vi "test.vi"() -> ()   [LabVIEW 2018]
doc: "This example demonstrates how to continuously acquire buffered voltage measurements using a DAQmx device.\n\nFor instructions on how to connect your signals to the DAQ device, refer to your device documentation."
uses:
  <vilib>/Utility/error.llb/DialogType.ctl
  <vilib>/DAQmx/read.llb/DAQmx Read (Analog 2D DBL NChan NSamp).vi
  <vilib>/Analysis/baseanly.llb/Mean (DBL).vi
  <vilib>/DAQmx/create/channels.llb/DAQmx Create Channel (AI-Voltage-Basic).vi
  <vilib>/DAQmx/configure/timing.llb/DAQmx Timing (Sample Clock).vi
  <vilib>/DAQmx/configure/task.llb/DAQmx Configure Logging (TDMS).vi
  <vilib>/DAQmx/configure/trigger.llb/DAQmx Start Trigger (Digital Edge).vi
  <vilib>/DAQmx/configure/trigger.llb/DAQmx Start Trigger (Time).vi
  <vilib>/DAQmx/configure/trigger.llb/DAQmx Start Trigger (Analog Edge).vi
  <vilib>/DAQmx/miscellaneous.llb/DAQmx Fill In Error Info.vi
  <resource>/objmgr/daqmx.rc
  <vilib>/Analysis/NI_AALBase.lvlib
panel:
  out "Numeric":i32
  out "Numeric 2":i32
  in  "SAVE":bool
  in  "Path":path
  in  "Name File":string
  in  "Trigger Type":T1(tab)=enum."Digital Start"
  in  "Digital Start Trigger Edge":i32(ring)=10280 caption="Edge" items=["Rising"=10280, "Falling"=10171]
  in  "Digital Start Trigger Source":tag="/Dev2/PFI0" caption="Source"
  in  "Digital Pause Trigger Pause When":i32(ring)=10192 caption="Pause When" items=["High"=10192, "Low"=10214]
  in  "Digital Pause Trigger Source":tag="/Dev1/PFI0" caption="Source"
  in  "Analog Start Trigger Level":dbl caption="Level" format="%0.2f"
  in  "Analog Start Trigger Hysteresis":dbl caption="Hysteresis" format="%.2f"
  in  "Analog Start Trigger Slope":i32(ring)=10280 caption="Slope" items=["Rising"=10280, "Falling"=10171]
  in  "Analog Start Trigger Source":string="APFI0" caption="Source"
  in  "Analog Pause Trigger Source":string="APFI0" caption="Source"
  in  "Analog Pause Trigger Pause When":i32(ring)=10093 caption="Pause When" items=["Above Level"=10093, "Below Level"=10107]
  in  "Analog Pause Trigger Level":dbl caption="Level" format="%.2f"
  in  "When":timestamp
  in  "Select Time\nManually":bool
  in  "SENSOR":bool
  out "Waveform Graph":dbl[][](graph)
  in  "TDMS File Path":path
  in  "Number of Samples":i32=100
  in  "Sample Rate":dbl=10000.0
  in  "Sample Clock Source":tag="OnboardClock"
  in  "Terminal Configuration":i32(ring)=10083 items=["default"=-1, "RSE"=10083, "NRSE"=10078, "Differential"=10106, "Pseudodifferential"=12529]
  in  "Max Voltage":dbl=10.0
  in  "Min Voltage":dbl=-10.0
  in  "Physical Channel":tag="Dev2/ai3:4"
  out "Actual Sample Rate":dbl=1000.0 format="%0.2f"
  in  "Logging Mode":i32(ring)=10231 items=["Off"=10231, "Log and Read"=15842]
  # "Channel Settings"
  # "Acquired Data"
  # "Timing Settings"
  # "Logging Settings"
  # "Trigger Settings"
  # "To enable triggers, select a tab above, and configure the settings.\n\nNot all hardware supports all trigger types. Refer to your device documentation for more information."
  # "This trigger type is not supported in continuous sample timing. \n\nRefer to your device documentation for more information on which triggers are supported."
  # "This trigger type is not supported in continuous sample timing. \n\nRefer to your device documentation for more information on which triggers are supported."
  # "If time is not manually set, task will begin after 10 seconds"
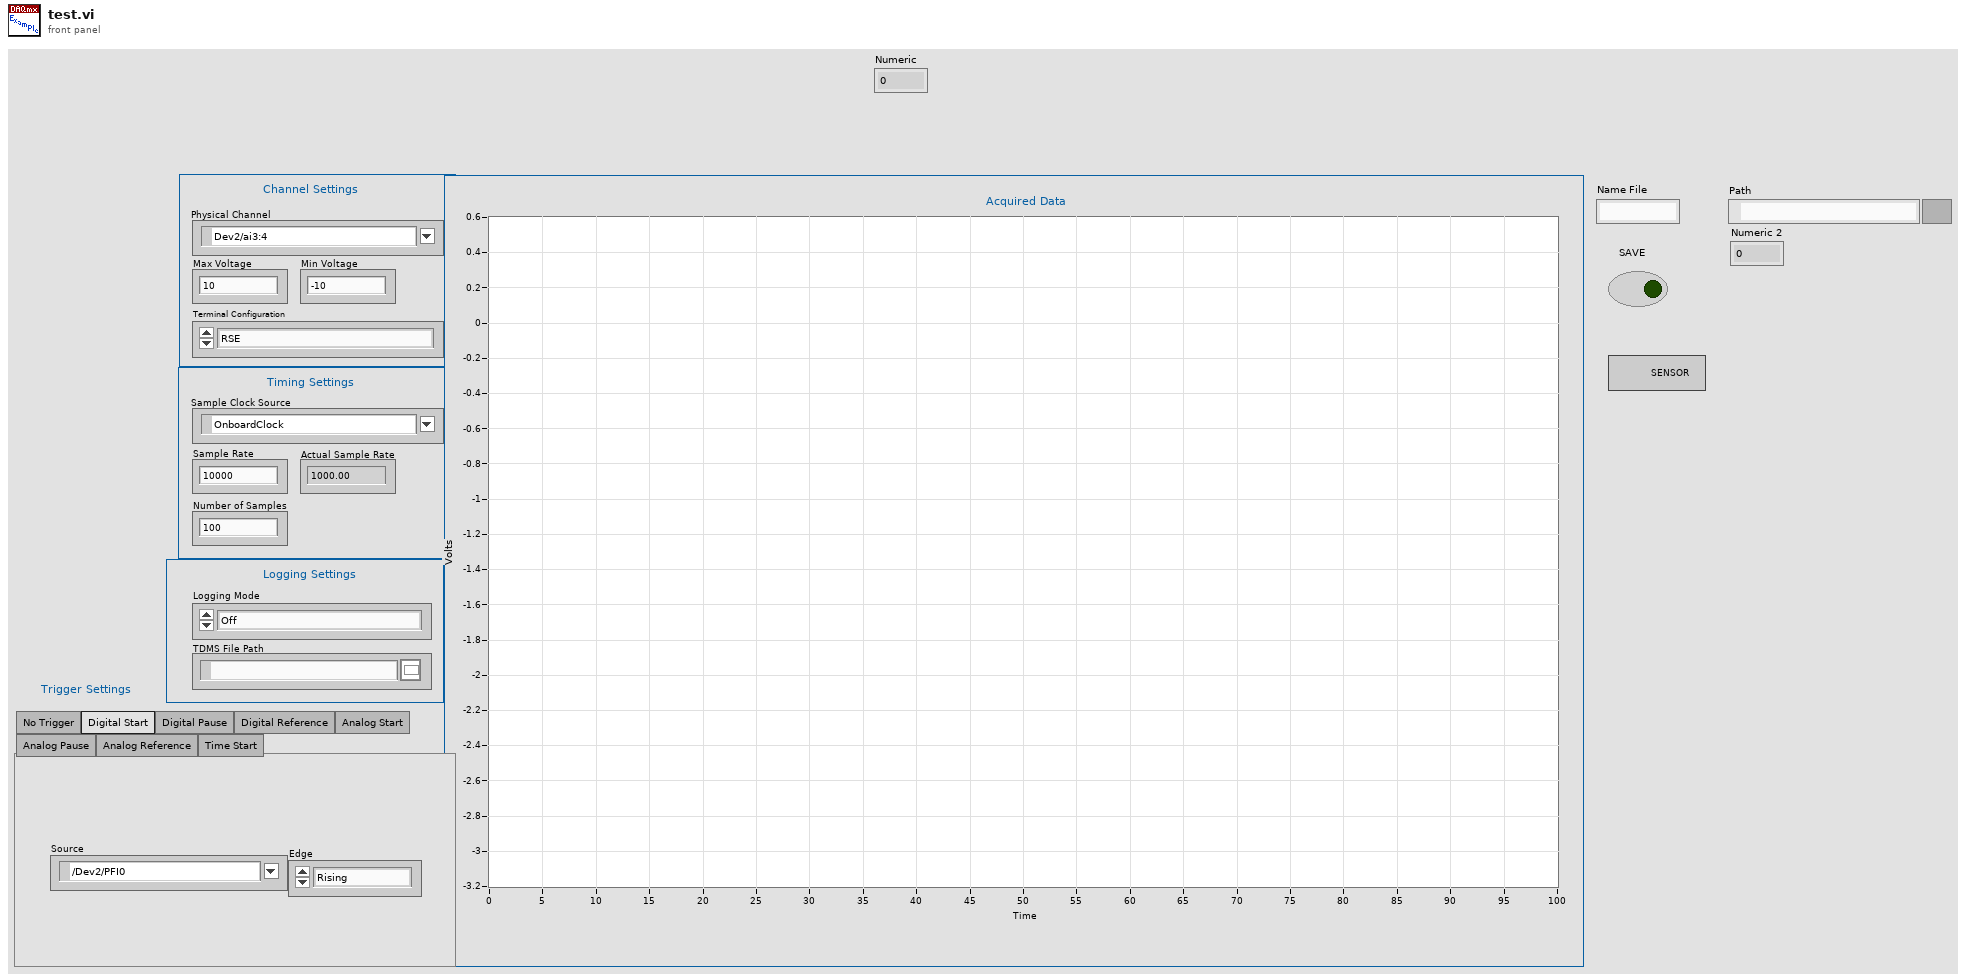
[diagram p1: front panel]
types:
  T1 = enum32{"No Trigger", "Digital Start", "Digital Pause", "Digital Reference", "Analog Start", "Analog Pause", "Analog Reference", "Time Start"}
  T2 = typedef "DialogType.ctl" = u16
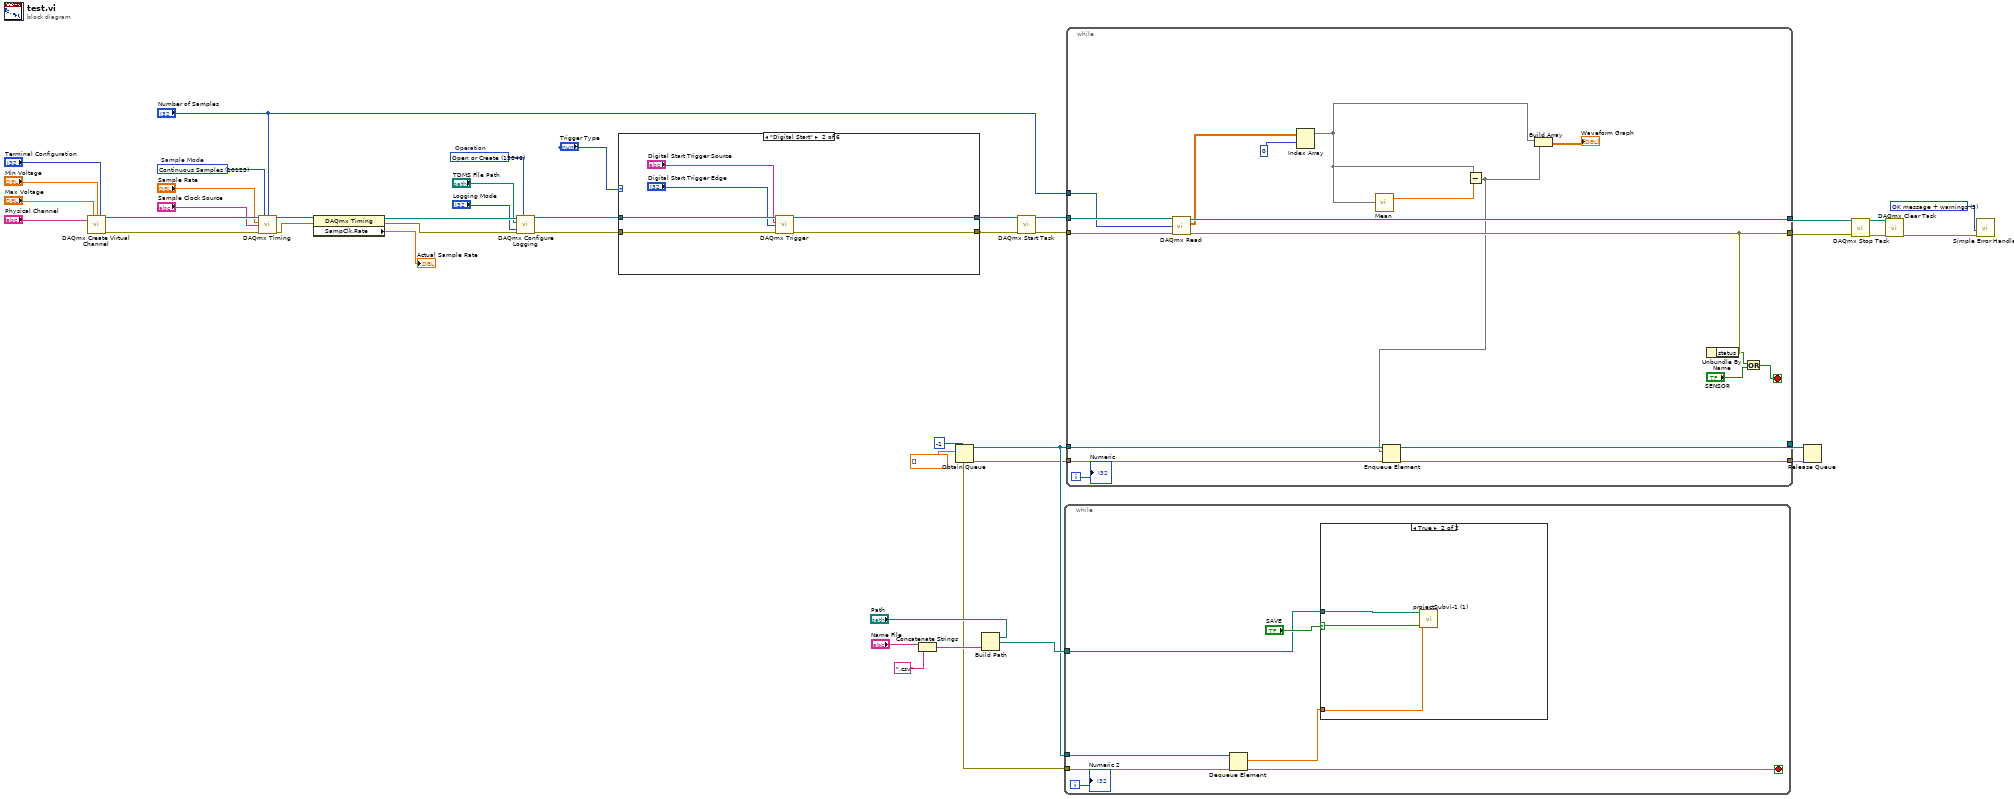
[diagram p0: block diagram]
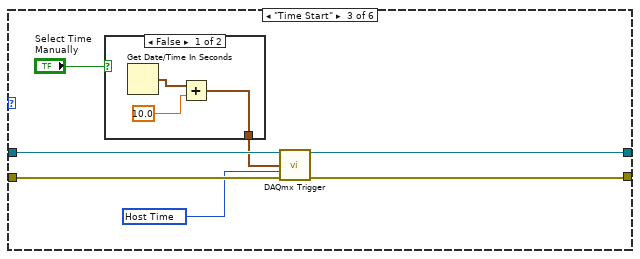
[diagram p4: hidden frame]
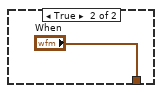
[diagram p5: hidden frame]
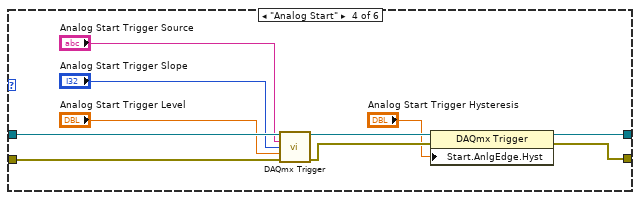
[diagram p6: hidden frame]
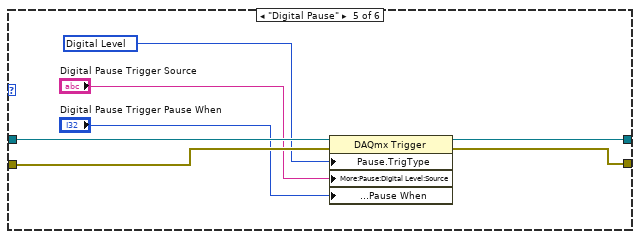
[diagram p7: hidden frame]
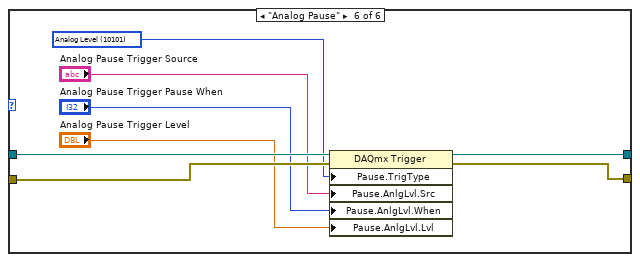
[diagram p8: hidden frame]
diagram:
  w17 = T2 3 items=["no dialog", "OK message", "continue or stop message", "OK message + warnings", "continue/stop + warnings"] ("type of dialog (OK msg:1)")
  w35 = 15846 items=["Open"=10437, "Open or Create"=15846, "Create or Replace"=15847, "Create"=15848]  # Operation
  w40 = 10123 items=["Finite Samples"=10178, "Continuous Samples"=10123, "Hardware Timed Single Point"=12522]  # Sample Mode
  n1 = call-poly <vilib>:"DAQmx Create Virtual Channel.vi"("maximum value"="Max Voltage", "minimum value"="Min Voltage", "input terminal configuration"="Terminal Configuration", "physical channels"="Physical Channel") -> ("task out"=w38:refnum<k21>, "error out"=w39:errorcluster)  [unwired: 10 in]
  n2 = call-poly <vilib>:"DAQmx Timing.vi"("task/channels in"=w38, "sample mode"=w40, "samples per channel"="Number of Samples", "rate"="Sample Rate", "source"="Sample Clock Source", "error in"=w39) -> ("task out"=w42:refnum<k21>, "error out"=w41:errorcluster)  [unwired: 8 in]
  n3 = property class="DAQmx Timing"(reference=w42, error in=w41) -> (reference out=w37:refnum<k21>, error out=w36:errorcluster, "SampClk.Rate"=→"Actual Sample Rate":dbl)
  n4 = call-poly <vilib>:"DAQmx Configure Logging.vi"("task/channels in"=w37, "operation"=w35, "file path"="TDMS File Path", "logging mode"="Logging Mode", "error in"=w36) -> ("task out"=w15:refnum<k21>, "error out"=w14:errorcluster)  [unwired: 9 in]
  n5 = case shown="\"Digital Start\"" "Trigger Type" {
    tunnel: w15 -> [w44 w50 w57 w71 w78 w86]
    tunnel: w14 -> [w43 w49 w56 w70 w75 w83]
    tunnel: [w44 w48 w55 w68 w77 w85] -> w12
    tunnel: [w43 w47 w54 w67 w76 w84] -> w13
    frame "No Trigger", Default {
    }
    frame "Digital Start" {
      n6 = call-poly <vilib>:"DAQmx Trigger.vi"("task/channels in"=w50, "source"="Digital Start Trigger Source", "edge"="Digital Start Trigger Edge", "error in"=w49) -> ("task out"=w48:refnum<k21>, "error out"=w47:errorcluster)  [unwired: 10 in]
    }
    frame "Time Start" {
      w53 = 16126 items=["Host Time"=16126, "I/O Device Time"=16127] ("timescale")
      n7 = case shown="False" "Select Time\nManually" {
        tunnel: [w58 "When"] -> w51
        frame False {
          n8 = Get Date/Time In Seconds() -> (seconds since 1Jan1904=w60:timestamp)
          n9 = Add(x=w60, y=10.0) -> (x+y=w58:timestamp)
        }
        frame True {
        }
      }
      n10 = call-poly <vilib>:"DAQmx Trigger.vi"("task/channels in"=w57, "when"=w51, "timescale"=w53, "error in"=w56) -> ("task out"=w55:refnum<k21>, "error out"=w54:errorcluster)  [unwired: 10 in]
    }
    frame "Analog Start" {
      n11 = call-poly <vilib>:"DAQmx Trigger.vi"("task/channels in"=w71, "source"="Analog Start Trigger Source", "slope"="Analog Start Trigger Slope", "level"="Analog Start Trigger Level", "error in"=w70) -> ("task out"=w66:refnum<k21>, "error out"=w65:errorcluster)  [unwired: 9 in]
      n12 = property class="DAQmx Trigger"(reference=w66, error in=w65, "Start.AnlgEdge.Hyst"="Analog Start Trigger Hysteresis") -> (reference out=w68:refnum<k21>, error out=w67:errorcluster)
    }
    frame "Digital Pause" {
      w74 = 10152 items=["Analog Level"=10101, "Analog Window"=10103, "Digital Level"=10152, "Digital Pattern"=10398, "None"=10230] ("Pause.TrigType")
      n13 = property class="DAQmx Trigger"(reference=w78, error in=w75, "Pause.TrigType"=w74, "More:Pause:Digital Level:Source"="Digital Pause Trigger Source", "More:Pause:Digital Level:Pause When"="Digital Pause Trigger Pause When") -> (reference out=w77:refnum<k21>, error out=w76:errorcluster)
    }
    frame "Analog Pause" {
      w82 = 10101 items=["Analog Level"=10101, "Analog Window"=10103, "Digital Level"=10152, "Digital Pattern"=10398, "None"=10230] ("Pause.TrigType")
      n14 = property class="DAQmx Trigger"(reference=w86, error in=w83, "Pause.TrigType"=w82, "Pause.AnlgLvl.Src"="Analog Pause Trigger Source", "Pause.AnlgLvl.When"="Analog Pause Trigger Pause When", "Pause.AnlgLvl.Lvl"="Analog Pause Trigger Level") -> (reference out=w85:refnum<k21>, error out=w84:errorcluster)
    }
  }
  n15 = Concatenate Strings("Name File", ".csv" ("string")) -> (w5:string)
  n16 = Obtain Queue(max queue size (-1, unlimited)=-1, element data type=dbl[] [] ("Radar output")) -> (queue out=w2:refnum<queue>, error out=w1:errorcluster)  [unwired: 3 in, 1 out]
  n17 = Build Path(base path="Path", name or relative path=w5) -> (appended path=w3:path)
  n18 = call <vilib>:"DAQmx Start Task.vi"("task/channels in"=w12, "error in"=w13) -> ("task out"=w34:refnum<k21>, "error out"=w33:errorcluster)  [unwired: 12 in]
  n19 = while {
    tunnel: w2 -> [w93]
    tunnel: w1 -> [w92]
    tunnel: w3 -> [w88]
    i -> [w87]
    stop <- w91 stop-if-true
    n20 = Dequeue Element(queue=w93, error in (no error)=w92) -> (element=w89:dbl[], error out=w91:errorcluster)  [unwired: 1 in, 2 out]
    n21 = case shown="True" "SAVE" {
      selector: "SAVE" -> [_ w94]
      tunnel: w89 -> [_ w95]
      tunnel: w88 -> [_ w96]
      frame False {
      }
      frame True {
        n22 = call "projectSubvi-1 (1).vi"("append to file? (new file:F)"=w94, "1D data"=w95, "file path (dialog if empty)"=w96) -> ()  [unwired: 9 in]
      }
    }
    "Numeric 2" <- w87
  }
  n23 = while {
    tunnel: w34 -> [w115]
    tunnel: w33 -> [w114]
    tunnel: [w113] -> w21
    tunnel: [w111] -> w20
    tunnel: "Number of Samples" -> [w109]
    tunnel: [w107] -> w11
    tunnel: [w106] -> w10
    tunnel: w2 -> [w105]
    tunnel: w1 -> [w104]
    i -> [w100]
    stop <- w99 stop-if-true
    n24 = call-poly <vilib>:"DAQmx Read.vi"("task/channels in"=w115, "number of samples per channel"=w109, "error in"=w114) -> ("task out"=w113:refnum<k21>, "data"=w103:dbl[][], "error out"=w111:errorcluster)  [unwired: 10 in]
    n25 = Index Array(array=w103, index (row)=0) -> (element=w101:dbl[])  [unwired: 1 in]
    n26 = call-poly <vilib>:"Mean.vi"("X"=w101) -> ("mean"=w102:dbl)  [unwired: 1 out]
    n27 = Subtract(x=w101, y=w102) -> (x-y=w97:dbl[])
    n28 = Enqueue Element(queue=w105, element=w97, error in (no error)=w104) -> (queue out=w107:refnum<queue>, error out=w106:errorcluster)  [unwired: 1 in, 1 out]
    n29 = Build Array(w101, w97) -> (→"Waveform Graph":dbl[][])
    n30 = Unbundle By Name(w111) -> ("status"=w110:bool)
    n31 = Or(x=w110, y="SENSOR") -> (x .or. y?=w99:bool)
    "Numeric" <- w100
  }
  n32 = Release Queue(queue=w11, error in (no error)=w10) -> ()  [unwired: 1 in, 3 out]
  n33 = call <vilib>:"DAQmx Stop Task.vi"("task/channels in"=w21, "error in"=w20) -> ("task out"=w18:refnum<k21>, "error out"=w19:errorcluster)  [unwired: 12 in]
  n34 = call <vilib>:"DAQmx Clear Task.vi"("task in"=w18, "error in"=w19) -> ("error out"=w32:errorcluster)  [unwired: 13 in]
  n35 = call <vilib>:"Simple Error Handler.vi"("type of dialog (OK msg:1)"=w17, "error in (no error)"=w32) -> ()  [unwired: 3 in, 5 out]
